vi "set_size.vi"(8 "error in (no error)":errorcluster, 10 "size":refnum<class "SpaceVector.lvclass">, 11 "RoiGeneric in":refnum<class "RoiGeneric.lvclass">) -> (0 "error out":errorcluster, 3 "RoiGeneric out":refnum<class "RoiGeneric.lvclass">)   [LabVIEW 2010, in "RoiGeneric.lvclass"]
uses:
  RoiGeneric.lvclass
  common/classes/SpaceVector/SpaceVector/SpaceVector.lvclass
  RoiGeneric.lvclass/RoiGeneric.ctl
  common/classes/Box/Box/Box.lvclass
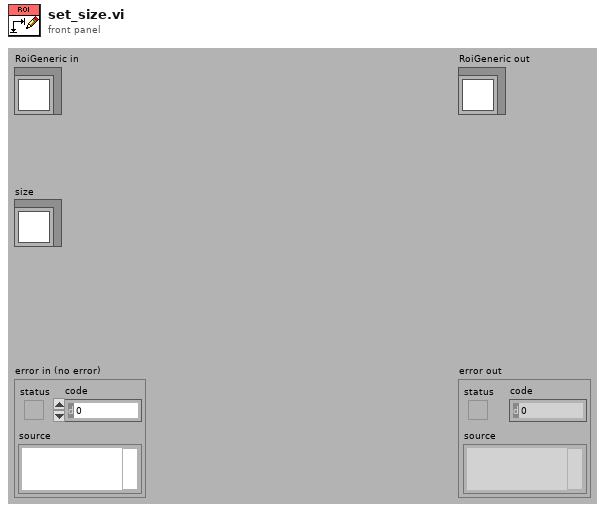
[diagram p1: front panel]
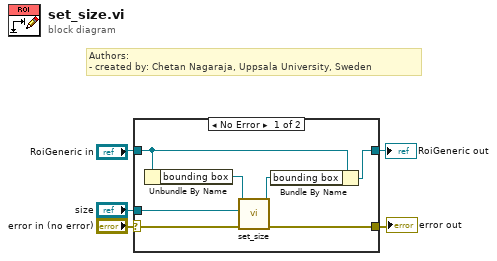
[diagram p0: block diagram]
diagram:
  # "Authors: \n- created by: Chetan Nagaraja, Uppsala University, Sweden"
  n1 = case shown="No Error" "error in (no error)" {
    selector: "error in (no error)" -> [w12 w14]
    tunnel: [w11 w14] -> w4
    tunnel: [w7 w13] -> w2
    tunnel: "RoiGeneric in" -> [w8 w13]
    tunnel: "size" -> [w6 _]
    frame No Error {
      n2 = Unbundle By Name(w8) -> ("bounding box"=w10:refnum<class "Box.lvclass">)
      n3 = call "set_size.vi"("error in (no error)"=w12, "new size"=w6, "Box in"=w10) -> ("error out"=w11:errorcluster, "Box out"=w9:refnum<class "Box.lvclass">)  [unwired: 7 in]
      n4 = Bundle By Name(cluster=w8, "bounding box"=w9) -> (w7:refnum<class "RoiGeneric.lvclass">)
    }
    frame Error {
    }
  }
  "error out" <- w4
  "RoiGeneric out" <- w2
